vi "global_vars.vi"() -> ()   [LabVIEW 2011]
panel:
  in  "UL_#Phase Shifts":i32
  in  "window size":cluster{"x Width(Px)":i32, "y height(Px)":i32}
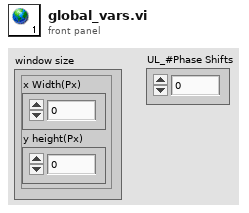
[diagram p1: front panel]
diagram:
